vi "write sequential Array of U32s.vi"(9 "values":cluster{"Array":u32[]}[](array[cluster]), 10 "index":i32, 11 "data table in":T1) -> (3 "data table out":T1)   [LabVIEW 2013, in "tag bus.lvlib" / "data table.lvlib"]
doc: "Writes a sequential set of data to the table."
uses:
  data table.lvlib
  data table.ctl
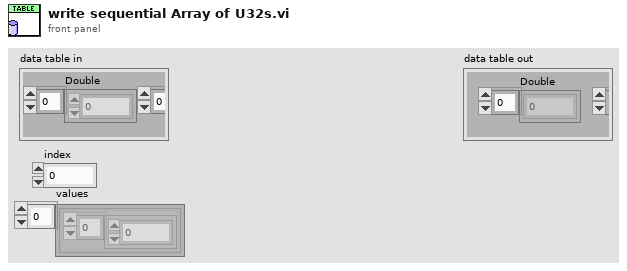
[diagram p1: front panel]
types:
  T1 = typedef "tag bus.lvlib/data table.lvlib/data table.ctl" = cluster{"Double":dbl[], "Single":sgl[], "I64":i64[], "I32":i32[], "I16":i16[], "I8":i8[], "U64":u64[], "U32":u32[], "U16":u16[], "U8":u8[], "Boolean":bool[], "String":string[], "Array of Double":cluster{"DBL Array":dbl[]}[], "Array of Single":cluster{"SGL Array":sgl[]}[], "Array of I64":cluster{"I64 Array":i64[]}[], "Array of I32":cluster{"I32 Array":i32[]}[], "Array of I16":cluster{"I16 Array":i16[]}[], "Array of I8":cluster{"I8 Array":i8[]}[], "Array of U64":cluster{"U64 Array":u64[]}[], "Array of U32":cluster{"U32 Array":u32[]}[], "Array of U16":cluster{"U16 Array":u16[]}[], "Array of U8":cluster{"U8 Array":u8[]}[], "Array of Boolean":cluster{"Boolean Array":bool[]}[], "Array of String":cluster{"String Array":string[]}[]}
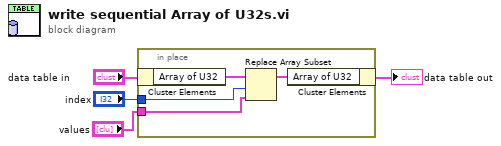
[diagram p0: block diagram]
diagram:
  n1 = in-place {
    in-place-border: "values" -> [w6]
    in-place-border: "index" -> [w5]
    n2 = in-place-cluster #1("data table in") -> ("Array of U32"=w8:cluster{"U32 Array":u32[]}[])
    n3 = Replace Array Subset(array=w8, new element=w6, index=w5) -> (w7:cluster{"U32 Array":u32[]}[])
    n4 = in-place-cluster #1("Array of U32"=w7) -> (→"data table out":T1)
  }
